vi "Handle Connections Value Change.vi"(4 "State":string, 7 "Channel Editor State":T1={"Modules and Connections"=[{" Module Path"="", "Short Module Path"="", "Product Name"="", "Possible Connections"=[], "Missing"=FALSE}, {" Module Path"="", "Short Module Path"="", "Product Name"="", "Possible Connections"=[], "Missing"=FALSE}], "Alias Mappings UI"=[], "Mappings by Module UI"=[]}, 8 "error in (no error)":errorcluster, 9 "OldVal":T7[](array[typedef]), 10 "NewVal":T7[](array[typedef]), 11 "Routing Channel Ref in":T8 format="%.0x") -> (0 "error out":errorcluster, 3 "Routing Channel Ref out":T8 format="%.0x")   [LabVIEW 2020, in "Routing and Faulting System Explorer.lvlib"]
uses:
  Routing and Faulting System Explorer.lvlib
  <vilib>/NI VeriStand/Custom Device API/Custom Device Item Ref.ctl
  Connection Row.ctl
  Channel Editor State.ctl
  Possible Connections.ctl
  Shared/Routing and Faulting Hardware API/Types/Possible Connections for Endpoint.ctl
  Shared/Alias Mapping.ctl
  Shared/Alias Endpoint.ctl
  Alias Map by Module.ctl
  e32bcdcd-e61b-4a24-afe7-32b08c6141fc.vi
  Scripting/Routing and Faulting Scripting.lvlib
  <vilib>/NI VeriStand/Custom Device API/Custom Device API.lvlib
  Shared/Routing and Faulting Shared.lvlib
  Shared/Routing and Faulting Hardware API/Routing and Faulting Hardware API.lvlib
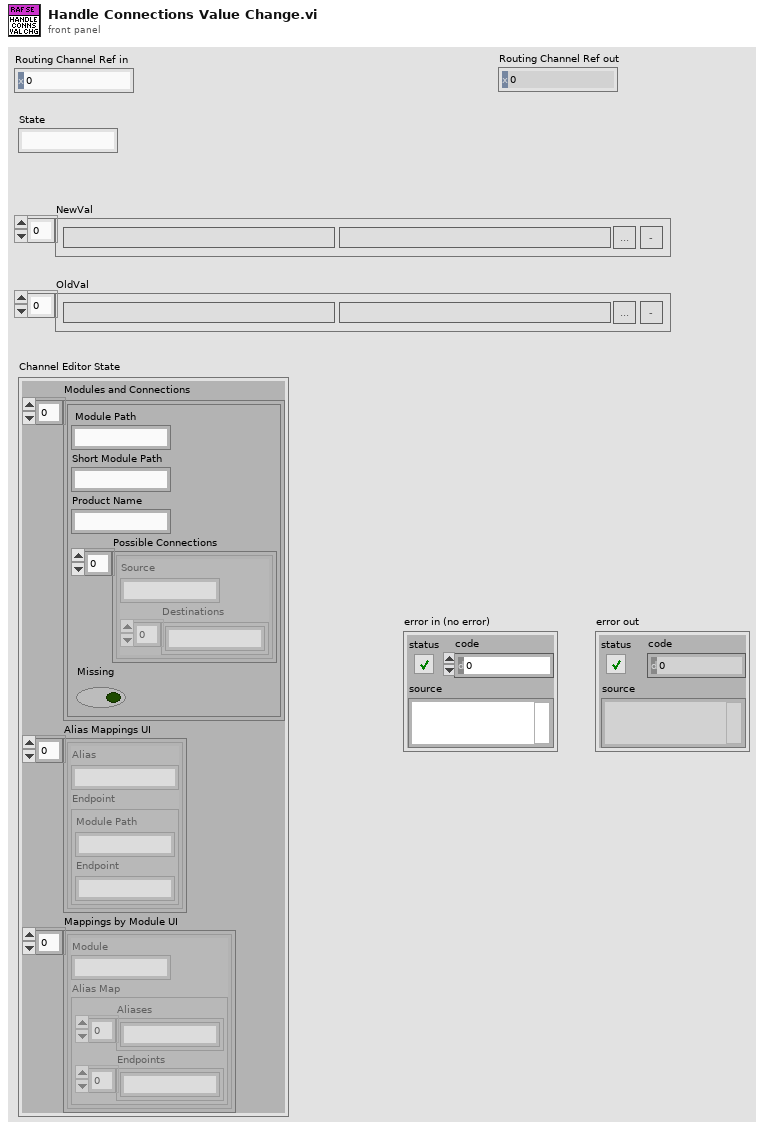
[diagram p1: front panel]
types:
  T1 = typedef "Routing and Faulting System Explorer.lvlib/Channel Editor State.ctl" = cluster{"Modules and Connections":T2[], "Alias Mappings UI":T4[], "Mappings by Module UI":T6[]}
  T2 = typedef "Routing and Faulting System Explorer.lvlib/Possible Connections.ctl" = cluster{" Module Path":string, "Short Module Path":string, "Product Name":string, "Possible Connections":T3[], "Missing":bool}
  T3 = typedef "Routing and Faulting Hardware API.lvlib/Possible Connections for Endpoint.ctl" = cluster{"Source":string, "Destinations":string[]}
  T4 = typedef "Routing and Faulting Shared.lvlib/Alias Mapping.ctl" = cluster{"Alias":string, "Endpoint":T5}
  T5 = typedef "Routing and Faulting Shared.lvlib/Alias Endpoint.ctl" = cluster{"Module Path":string, "Endpoint":string}
  T6 = typedef "Routing and Faulting System Explorer.lvlib/Alias Map by Module.ctl" = cluster{"Module":string, "Alias Map":cluster{"Aliases":string[], "Endpoints":string[]}}
  T7 = typedef "Routing and Faulting System Explorer.lvlib/Connection Row.ctl" = cluster{"Source":string, "Destination":string, "Edit":bool, "Remove":bool}
  T8 = typedef "Custom Device API.lvlib/Custom Device Item Ref.ctl" = u64
  T9 = cluster{"Source":bool, "Destination":bool, "Edit":bool, "Remove":bool}
  T10 = typedef "Routing and Faulting Shared.lvlib/Connection.ctl" = cluster{"Module":string, "Source":string, "Destination":string}
  T11 = typedef "Routing and Faulting Shared.lvlib/Routing State.ctl" = cluster{"Name":string, "Description":string, "Value":i32, "Connection List":T10[]}
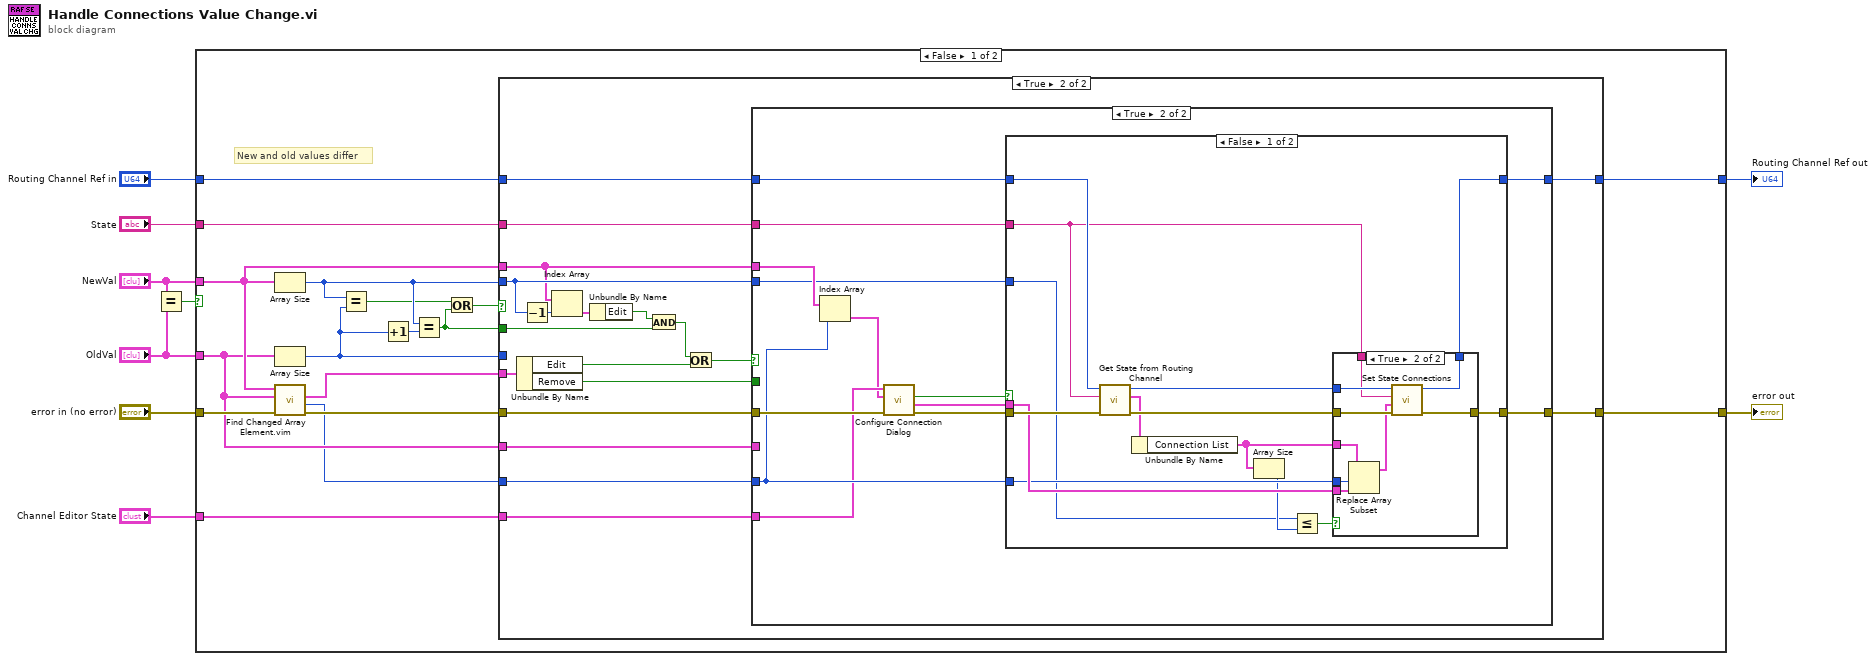
[diagram p0: block diagram]
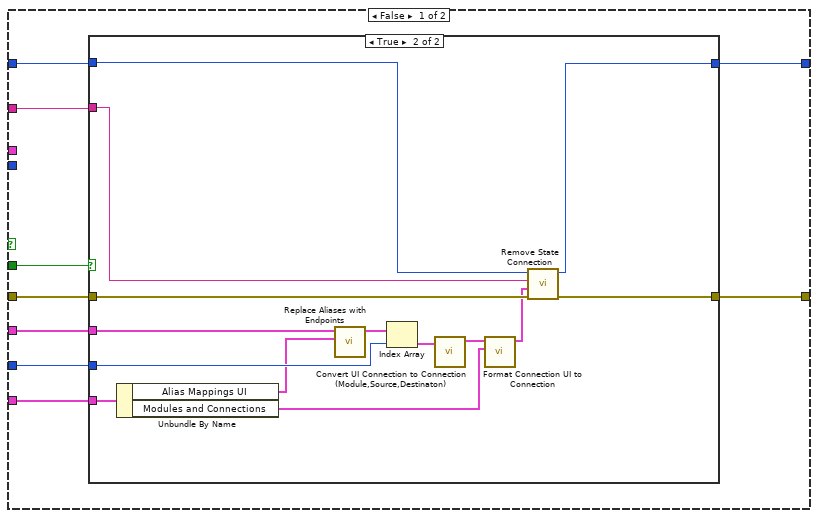
[diagram p3: hidden frame]
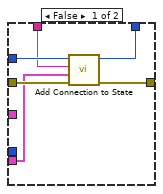
[diagram p5: hidden frame]
diagram:
  n1 = Equal?(x="NewVal", y="OldVal") -> (x = y?=w5:bool)
  n2 = case shown="False" w5 {
    tunnel: "error in (no error)" -> [w26 w117]
    tunnel: "Routing Channel Ref in" -> [w24 w118]
    tunnel: "NewVal" -> [w23 _]
    tunnel: "OldVal" -> [w22 _]
    tunnel: [w20 w117] -> w7
    tunnel: [w19 w118] -> w6
    tunnel: "State" -> [w17 _]
    tunnel: "Channel Editor State" -> [w10 _]
    frame False {
      # "New and old values differ"
      n3 = Array Size(array=w23) -> (size(s)=w14:i32)
      n4 = Array Size(array=w22) -> (size(s)=w16:i32)
      n5 = call "Find Changed Array Element.vim"("error in (no error)"=w26, "OldVal"=w22, "NewVal"=w23) -> ("error out"=w21:errorcluster, "Array Index"=w18:i32, "Element Changed"=w25:T9)  [unwired: 6 in]
      n6 = Equal?(x=w14, y=w16) -> (x = y?=w12:bool)
      n7 = Increment(x=w16) -> (x+1=w15:i32)
      n8 = Equal?(x=w14, y=w15) -> (x = y?=w11:bool)
      n9 = Or(x=w12, y=w11) -> (x .or. y?=w13:bool)
      n10 = case shown="True" w13 {
        tunnel: w18 -> [_ w41]
        tunnel: w25 -> [_ w47]
        tunnel: w14 -> [_ w36]
        tunnel: w16 -> [_ _]
        tunnel: w24 -> [w28 w45]
        tunnel: w23 -> [_ w34]
        tunnel: w22 -> [_ w46]
        tunnel: w21 -> [w27 w42]
        tunnel: [w27 w44] -> w20
        tunnel: [w28 w43] -> w19
        tunnel: w17 -> [_ w40]
        tunnel: w11 -> [_ w31]
        tunnel: w10 -> [_ w29]
        frame False {
          # "This case can happen if items are inserted or removed from the array\nshortcut menu during runtime. This is a lot of extra code to handle,\nso the shortcut menu for the Connections array is\ncurrently disabled to prevent this code path.\nIf the shortcut menu is ever re-enabled, code for handling add/remove\nshould go in this case."
        }
        frame True {
          n11 = Unbundle By Name(w47) -> ("Edit"=w39:bool, "Remove"=w38:bool)
          n12 = Decrement(x=w36) -> (x-1=w35:i32)
          n13 = Index Array(array=w34, index=w35) -> (element=w33:T7)
          n14 = Unbundle By Name(w33) -> ("Edit"=w32:bool)
          n15 = And(x=w32, y=w31) -> (x .and. y?=w30:bool)
          n16 = Or(x=w30, y=w39) -> (x .or. y?=w37:bool)
          n17 = case shown="True" w37 {
            tunnel: w46 -> [w56 _]
            tunnel: w45 -> [w55 w85]
            tunnel: [w54 w80] -> w44
            tunnel: [w53 w79] -> w43
            tunnel: w42 -> [w52 w84]
            tunnel: w34 -> [_ w77]
            tunnel: w41 -> [w51 w81]
            tunnel: w40 -> [w50 w78]
            tunnel: w38 -> [w49 _]
            tunnel: w36 -> [_ w76]
            tunnel: w29 -> [w48 w75]
            frame False {
              n18 = case shown="True" w49 {
                tunnel: w51 -> [_ w64]
                tunnel: w55 -> [w58 w70]
                tunnel: w56 -> [_ w72]
                tunnel: w52 -> [w57 w69]
                tunnel: [w57 w66] -> w54
                tunnel: [w58 w68] -> w53
                tunnel: w50 -> [_ w65]
                tunnel: w48 -> [_ w63]
                frame False {
                }
                frame True {
                  n19 = Unbundle By Name(w63) -> ("Alias Mappings UI"=w62:T4[], "Modules and Connections"=w59:T2[])
                  n20 = call "Replace Aliases with Endpoints.vi"("Alias Mappings"=w62, "UI Connections List in"=w72) -> ("UI Connections List out"=w67:T7[])  [unwired: 9 in]
                  n21 = Index Array(array=w67, index=w64) -> (element=w71:T7)
                  n22 = call "Convert UI Connection to Connection (Module,Source,Destinaton).vi"("Connection"=w71) -> ("Connection (Module,Source,Destinaton)"=w61:T10)  [unwired: 10 in]
                  n23 = call "Format Connection UI to Connection.vi"("Modules and Connections"=w59, "Connection UI"=w61) -> ("Connection"=w60:T10)  [unwired: 9 in]
                  n24 = call "Remove State Connection.vi"("error in"=w69, "connection"=w60, "state"=w65, "routing channel in"=w70) -> ("error out"=w66:errorcluster, "routing channel out"=w68:T8)  [unwired: 6 in]
                }
              }
            }
            frame True {
              n25 = Index Array(array=w77, index=w81) -> (element=w74:T7)
              n26 = call "Configure Connection Dialog.vi"("error in (no error)"=w84, "Current Connection"=w74, "Channel Editor State"=w75) -> ("error out"=w83:errorcluster, "Connection (R,S,D)"=w73:T10, "Canceled?"=w82:bool)  [unwired: 6 in]
              n27 = case shown="False" w82 {
                tunnel: w85 -> [w98 w115]
                tunnel: w73 -> [w94 _]
                tunnel: w83 -> [w97 w116]
                tunnel: [w95 w116] -> w80
                tunnel: w81 -> [w92 _]
                tunnel: [w91 w115] -> w79
                tunnel: w78 -> [w90 _]
                tunnel: w76 -> [w86 _]
                frame False {
                  n28 = call "Get State from Routing Channel.vi"("error in"=w97, "state"=w90, "routing channel in"=w98) -> ("error out"=w96:errorcluster, "state and connections"=w93:T11, "routing channel out"=w99:T8)  [unwired: 6 in]
                  n29 = Unbundle By Name(w93) -> ("Connection List"=w89:T10[])
                  n30 = Array Size(array=w89) -> (size(s)=w88:i32)
                  n31 = Less Or Equal?(x=w86, y=w88) -> (x <= y?=w87:bool)
                  n32 = case shown="True" w87 {
                    tunnel: w99 -> [w105 w114]
                    tunnel: w96 -> [w104 w113]
                    tunnel: [w102 w112] -> w95
                    tunnel: w94 -> [w101 w111]
                    tunnel: w92 -> [_ w110]
                    tunnel: [w103 w108] -> w91
                    tunnel: w90 -> [w100 w107]
                    tunnel: w89 -> [_ w106]
                    frame False {
                      n33 = call "Add Connection to State.vi"("error in"=w104, "connection"=w101, "state"=w100, "routing channel in"=w105) -> ("error out"=w102:errorcluster, "routing channel out"=w103:T8)  [unwired: 6 in]
                    }
                    frame True {
                      n34 = Replace Array Subset(array=w106, new element=w111, index=w110) -> (w109:T10[])
                      n35 = call "Set State Connections.vi"("error in"=w113, "connections"=w109, "state"=w107, "routing channel in"=w114) -> ("error out"=w112:errorcluster, "routing channel out"=w108:T8)  [unwired: 6 in]
                    }
                  }
                }
                frame True {
                }
              }
            }
          }
        }
      }
    }
    frame True {
      # "New and old values are the same. Do nothing"
    }
  }
  "Routing Channel Ref out" <- w6
  "error out" <- w7
